vi "CVT_RT_PARAM.vi"(11 "Param":T2={"Common"={"Velocity range"={"output high"=29.0, "output low"=-29.0}, "Vel_BasePos"=5, "Ref.Load_FindBase_L"=2.0, "Ref.Load_FindBase_R"=2.0, "Force_Peak"=150.0}, "Param_Left"={"L_기준값"=90.0, "L_검출값"=120.0, "L_End %"=42, "L_Onset %"=4, "L_Peak %"=28, "L_Pos"=0, "L_Offset"=0.0}, "Param_Right"={"R_기준값"=90.0, "R_검출값"=120.0, "R_End %"=42, "R_Onset %"=4, "R_Peak %"=28, "R_Pos"=0, "R_Offset"=0.0}}) -> (3 "RT_Config":T1)   [LabVIEW 2023]
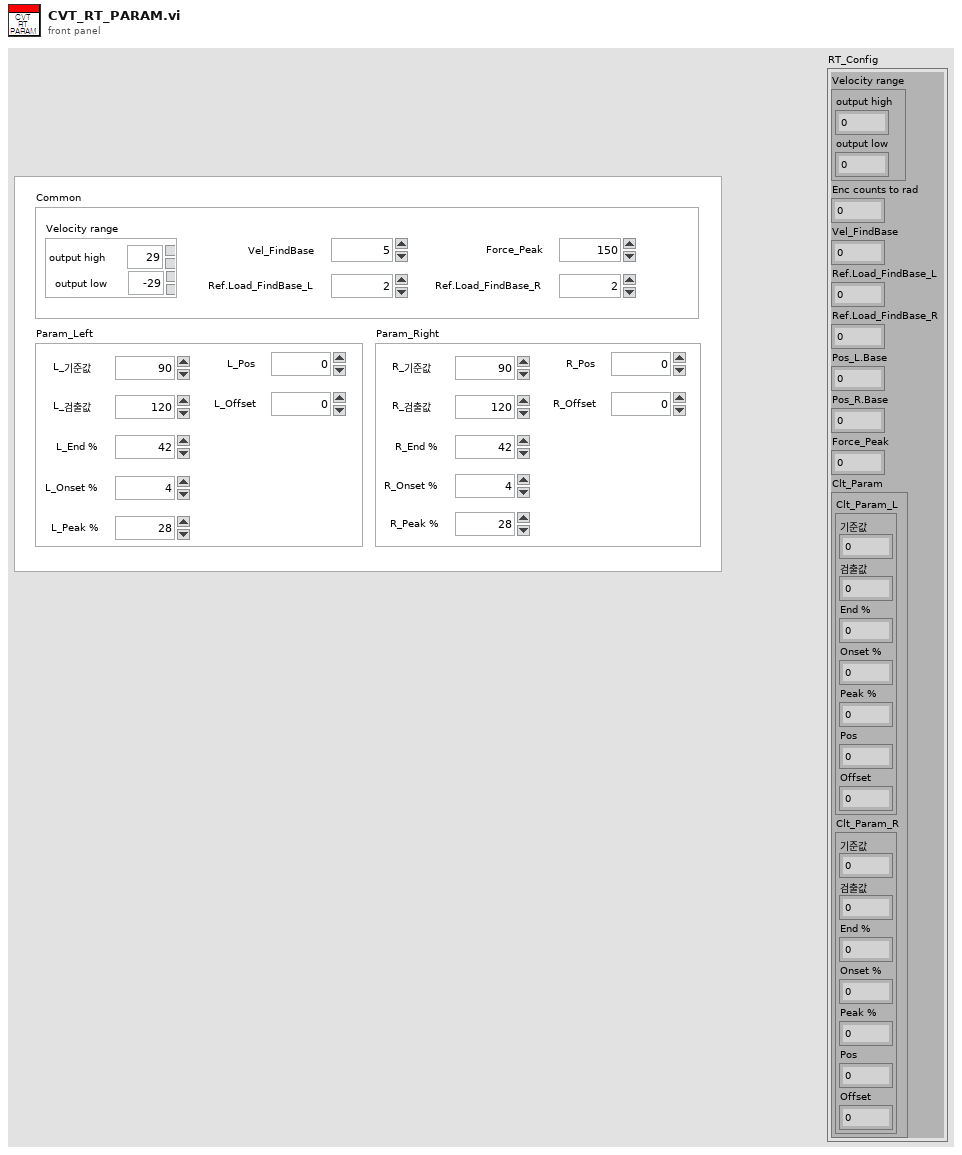
[diagram p1: front panel]
types:
  T1 = cluster{"Velocity range":cluster{"output high":dbl, "output low":dbl}, "Enc counts to rad":dbl, "Vel_FindBase":i32, "Ref.Load_FindBase_L":dbl, "Ref.Load_FindBase_R":dbl, "Pos_L.Base":dbl, "Pos_R.Base":dbl, "Force_Peak":dbl, "Clt_Param":cluster{"Clt_Param_L":cluster{"기준값":sgl, "검출값":sgl, "End %":i32, "Onset %":i32, "Peak %":i32, "Pos":i32, "Offset":sgl}, "Clt_Param_R":cluster{"기준값":sgl, "검출값":sgl, "End %":i32, "Onset %":i32, "Peak %":i32, "Pos":i32, "Offset":sgl}}}
  T2 = cluster{"Common":cluster{"Velocity range":cluster{"output high":dbl, "output low":dbl}, "Vel_BasePos":i32, "Ref.Load_FindBase_L":dbl, "Ref.Load_FindBase_R":dbl, "Force_Peak":dbl}, "Param_Left":cluster{"L_기준값":sgl, "L_검출값":sgl, "L_End %":i32, "L_Onset %":i32, "L_Peak %":i32, "L_Pos":i32, "L_Offset":sgl}, "Param_Right":cluster{"R_기준값":sgl, "R_검출값":sgl, "R_End %":i32, "R_Onset %":i32, "R_Peak %":i32, "R_Pos":i32, "R_Offset":sgl}}
  T3 = cluster{"L_기준값":sgl, "L_검출값":sgl, "L_End %":i32, "L_Onset %":i32, "L_Peak %":i32, "L_Pos":i32, "L_Offset":sgl}
  T4 = cluster{"R_기준값":sgl, "R_검출값":sgl, "R_End %":i32, "R_Onset %":i32, "R_Peak %":i32, "R_Pos":i32, "R_Offset":sgl}
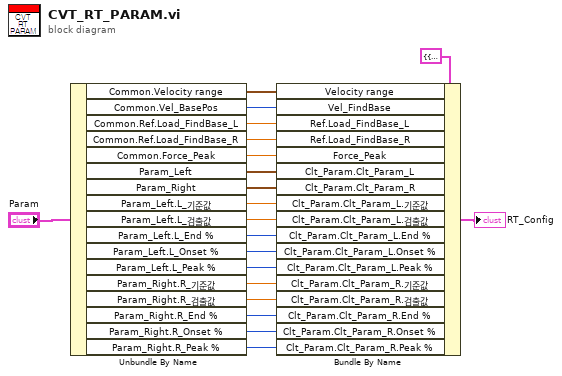
[diagram p0: block diagram]
diagram:
  n1 = Unbundle By Name("Param") -> ("Common.Velocity range"=w20:cluster{"output high":dbl, "output low":dbl}, "Common.Vel_BasePos"=w19:i32, "Common.Ref.Load_FindBase_L"=w18:dbl, "Common.Ref.Load_FindBase_R"=w17:dbl, "Common.Force_Peak"=w15:dbl, "Param_Left"=w14:T3, "Param_Right"=w13:T4, "Param_Left.L_기준값"=w12:sgl, "Param_Left.L_검출값"=w11:sgl, "Param_Left.L_End %"=w10:i32, "Param_Left.L_Onset %"=w9:i32, "Param_Left.L_Peak %"=w8:i32, "Param_Right.R_기준값"=w7:sgl, "Param_Right.R_검출값"=w6:sgl, "Param_Right.R_End %"=w5:i32, "Param_Right.R_Onset %"=w4:i32, "Param_Right.R_Peak %"=w3:i32)
  n2 = Bundle By Name(cluster=T1 {"Velocity range"={"output high"=0.0, "output low"=0.0}, "Enc counts to rad"=0.0, "Vel_FindBase"=0, "Ref.Load_FindBase_L"=0.0, "Ref.Load_FindBase_R"=0.0, "Pos_L.Base"=0.0, "Pos_R.Base"=0.0, "Force_Peak"=0.0, "Clt_Param"={"Clt_Param_L"={"기준값"=0.0, "검출값"=0.0, "End %"=0, "Onset %"=0, "Peak %"=0, "Pos"=0, "Offset"=0.0}, "Clt_Param_R"={"기준값"=0.0, "검출값"=0.0, "End %"=0, "Onset %"=0, "Peak %"=0, "Pos"=0, "Offset"=0.0}}} ("Param 2"), "Velocity range"=w20, "Vel_FindBase"=w19, "Ref.Load_FindBase_L"=w18, "Ref.Load_FindBase_R"=w17, "Force_Peak"=w15, "Clt_Param.Clt_Param_L"=w14, "Clt_Param.Clt_Param_R"=w13, "Clt_Param.Clt_Param_L.기준값"=w12, "Clt_Param.Clt_Param_L.검출값"=w11, "Clt_Param.Clt_Param_L.End %"=w10, "Clt_Param.Clt_Param_L.Onset %"=w9, "Clt_Param.Clt_Param_L.Peak %"=w8, "Clt_Param.Clt_Param_R.기준값"=w7, "Clt_Param.Clt_Param_R.검출값"=w6, "Clt_Param.Clt_Param_R.End %"=w5, "Clt_Param.Clt_Param_R.Onset %"=w4, "Clt_Param.Clt_Param_R.Peak %"=w3) -> (→"RT_Config":T1)
